vi "Add_User P3.vi"(8 "error in (no error)":errorcluster) -> (0 "error out":errorcluster)   [LabVIEW 2020]
uses:
  <vilib>/Utility/error.llb/DialogType.ctl
  <vilib>/Utility/file.llb/Write Delimited Spreadsheet (string).vi
  <vilib>/Utility/file.llb/Read Delimited Spreadsheet (string).vi
panel:
  in  "BACK TO MAIN":bool
  in  "Access Level":u16(ring) items=["User", "Super User", "Admin"]
  in  "User Control":string[][](table)
  in  "Save":bool
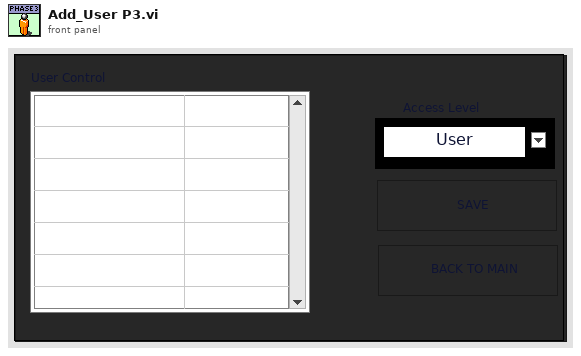
[diagram p1: front panel]
types:
  T1 = typedef "file folder ctl.ctl" = cluster{"Datalog path":path, "Configuration path":path, "Signal list path":path, "Sub vi's":path, "Authentication":path}
  T2 = typedef "LVRowAndColumnTypeDef.ctl" = cluster{"Row":i32, "Column":i32}
  T3 = typedef "DialogType.ctl" = u16
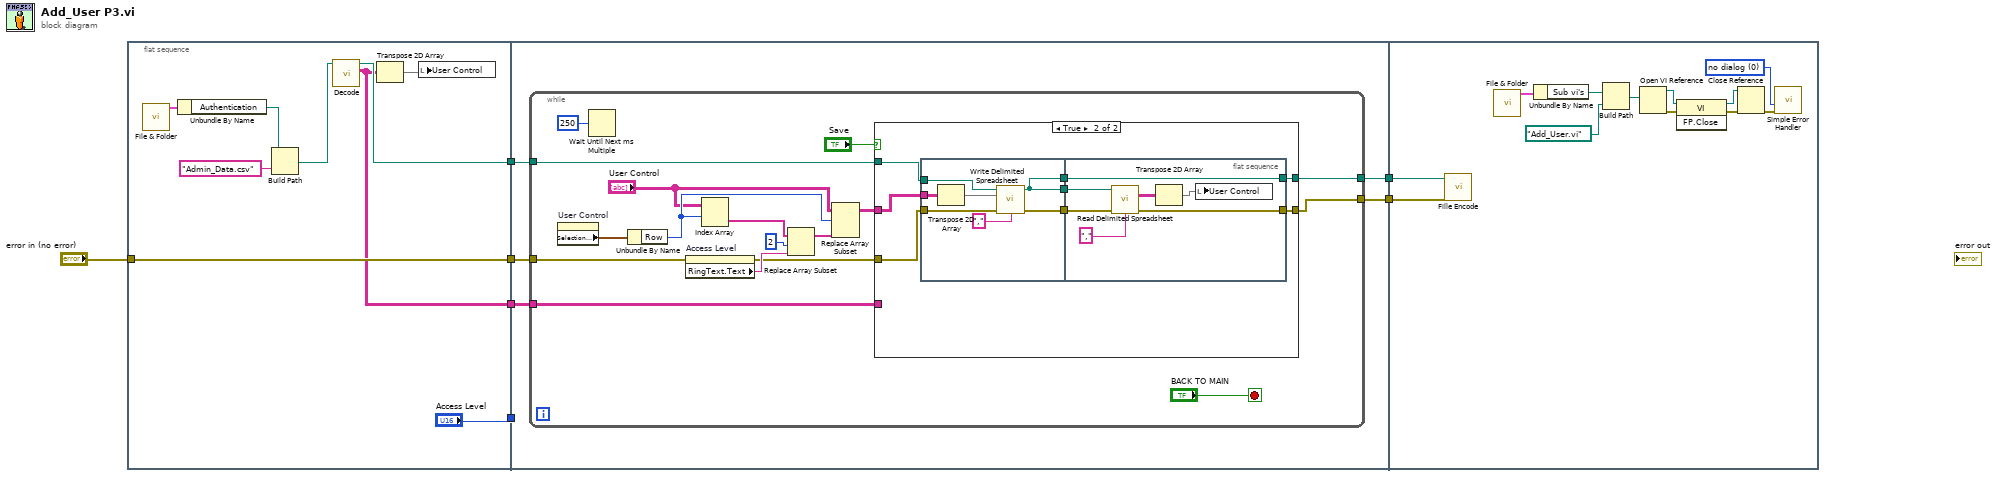
[diagram p0: block diagram]
diagram:
  n1 = flat-sequence {
    tunnel: ["Access Level"] -> w7
    tunnel: [w9] -> w6
    tunnel: "error in (no error)" -> [w14]
    tunnel: [w14] -> w5
    tunnel: [w8] -> w3
    tunnel: w7 -> [_]
    tunnel: w6 -> [w21]
    tunnel: w5 -> [w20]
    tunnel: w3 -> [w19]
    tunnel: [w18] -> w2
    tunnel: [w17] -> w1
    tunnel: w2 -> [w63]
    tunnel: w1 -> [w64]
    frame #0 {
      n2 = call "File & Folder.vi"() -> ("File Output"=w13:T1)  [unwired: 10 in, 1 out]
      n3 = Unbundle By Name(w13) -> ("Authentication"=w12:path)
      n4 = Build Path(base path=w12, name or relative path="Admin_Data.csv" ("name")) -> (appended path=w11:path)
      n5 = call "Decode.vi"("Encoded  File"=w11) -> ("array"=w8:string[][], "Decoded File"=w9:path)  [unwired: 9 in]
      n6 = Transpose 2D Array(2D array=w8) -> (transposed array=w10:string[][])
      n7 = local write "User Control"(w10) -> ()
    }
    frame #1 {
      n8 = while {
        tunnel: w21 -> [w25]
        tunnel: w20 -> [w28]
        tunnel: w19 -> [w24]
        tunnel: [w23] -> w18
        tunnel: [w22] -> w17
        stop <- "BACK TO MAIN" stop-if-true
        n9 = property on="User Control" class="Tbl (strict)"() -> ("Selection Start"=w38:T2)  [unwired: 2 in, 2 out]
        n10 = Wait Until Next ms Multiple(millisecond multiple=u32 250) -> ()  [unwired: 1 out]
        n11 = Unbundle By Name(w38) -> ("Row"=w36:i32)
        n12 = property on="Access Level" class="Ring (strict)"(error in=w28) -> (error out=w27:errorcluster, "RingText.Text"=w32:string)  [unwired: 1 in, 1 out]
        n13 = Index Array(array="User Control", index (row)=w36) -> (element=w35:string[])  [unwired: 1 in]
        n14 = Replace Array Subset(array=w35, new element=w32, index=2) -> (w33:string[])
        n15 = Replace Array Subset(array="User Control", new element=w33, index (row)=w36) -> (w37:string[][])  [unwired: 1 in]
        n16 = case shown="True" "Save" {
          tunnel: w37 -> [_ w44]
          tunnel: w25 -> [w40 w45]
          tunnel: w27 -> [w39 w46]
          tunnel: w24 -> [_ _]
          tunnel: [w40 w42] -> w22
          tunnel: [w39 w41] -> w23
          frame False {
          }
          frame True {
            n17 = flat-sequence {
              tunnel: w44 -> [w55]
              tunnel: w45 -> [w54]
              tunnel: [w49] -> w48
              tunnel: w46 -> [w52]
              tunnel: [w51] -> w47
              tunnel: [w49] -> w43
              tunnel: w48 -> [w62]
              tunnel: w47 -> [w60]
              tunnel: [w59] -> w41
              tunnel: [w56] -> w42
              tunnel: w43 -> [w56]
              frame #0 {
                n18 = Transpose 2D Array(2D array=w55) -> (transposed array=w50:string[][])
                n19 = call-poly <vilib>:"Write Delimited Spreadsheet.vi"("file path (dialog if empty)"=w54, "2D data"=w50, "error in (no error)"=w52, "delimiter (\\t)"="," ("delimiter (\\t)")) -> ("new file path (Not A Path if cancelled)"=w49:path, "error out"=w51:errorcluster)  [unwired: 10 in]
              }
              frame #1 {
                n20 = call-poly <vilib>:"Read Delimited Spreadsheet.vi"("file path (dialog if empty)"=w62, "error in (no error)"=w60, "delimiter (\\t)"="," ("delimiter (\\t)")) -> ("all rows"=w57:string[][], "error out"=w59:errorcluster)  [unwired: 7 in, 4 out]
                n21 = Transpose 2D Array(2D array=w57) -> (transposed array=w58:string[][])
                n22 = local write "User Control"(w58) -> ()
              }
            }
          }
        }
      }
    }
    frame #2 {
      w65 = T3 0 items=["no dialog", "OK message", "continue or stop message", "OK message + warnings", "continue/stop + warnings"] ("type of dialog (OK msg:1)")
      n23 = call "Fille Encode.vi"("error in"=w63, "Original File"=w64) -> ()  [unwired: 8 in, 2 out]
      n24 = call "File & Folder.vi"() -> ("File Output"=w72:T1)  [unwired: 10 in, 1 out]
      n25 = Unbundle By Name(w72) -> ("Sub vi's"=w71:path)
      n26 = Build Path(base path=w71, name or relative path=path "Add_User.vi") -> (appended path=w74:path)
      n27 = Open VI Reference(vi path=w74) -> (vi reference=w70:refnum<vi>, error out=w69:errorcluster)  [unwired: 5 in]
      n28 = invoke class="VI" method="FP.Close"(reference=w70, error in=w69) -> (reference out=w68:refnum<vi>, error out=w67:errorcluster)  [unwired: 1 in, 1 out]
      n29 = Close Reference(reference=w68, error in (no error)=w67) -> (error out=w66:errorcluster)
      n30 = call <vilib>:"Simple Error Handler.vi"("type of dialog (OK msg:1)"=w65, "error in (no error)"=w66) -> ()  [unwired: 3 in, 5 out]
    }
  }
